vi "Fdx Configure Rx VL Filter.vi"(8 "error in":errorcluster, 9 "VLControl":T1 {"FilterMode" items=["FDX_RX_VL_FLT_DIS", "FDX_RX_VL_FLT_ENA ", "FDX_RX_VL_FLT_ENA_INV"]; "VerificationMode" items=["FDX_RX_VL_CHECK_ENA_DEFAULT"=65535, "FDX_RX_VL_CHECK_REDMAM"=16, "DX_RX_VL_CHECK_TRAFIC"=8, "FDX_RX_VL_CHECK_FRAMESIZE"=4, "FDX_RX_VL_CHECK_SNINTEG"=2, "FDX_RX_VL_CHECK_INVPAC"=1, "FDX_RX_VL_CHECK_DISA"=0]; "PayloadMode" items=["FDX_PAYLOAD_FULL", "FDX_PAYLOAD_IP_EXT", "FDX_PAYLOAD_IP", "FDX_PAYLOAD_MAC"]; "EnableMode" items=["FDX_RX_VL_DIS "=0, "FDX_RX_VL_ENA_STAT"=1, "FDX_RX_VL_ENA_CNT "=2, "FDX_RX_VL_ENA_MON_ALL"=3, "FDX_RX_VL_ENA_MON_GOOD"=7, "FDX_RX_VL_ENA_EXT"=4]}, 11 "InstrumentHandle_port":u32) -> (0 "error out":errorcluster, 3 "InstrumentHandle_port":u32)   [LabVIEW 2020, in "AIM664LV.lvlib"]
doc: "This function is used to control the Virtual link specific setting for a receive port. The settings for a VL can be equivalent to a VL capture filter. That means, only data of a VL which is enabled for capturing, will be stored in the associated buffer."
uses:
  AIM664LV.lvlib
  AFDX_LibraryAdmin/FdxGlobalDllPath.vi
panel:
  # "Inputs"
  # "Outputs"
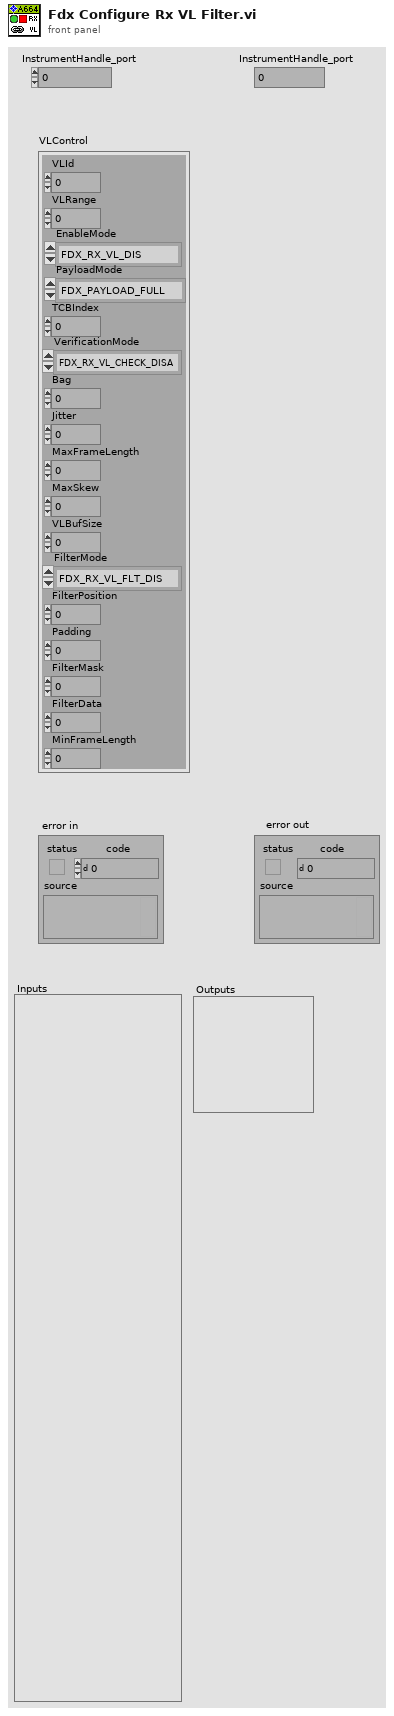
[diagram p1: front panel]
types:
  T1 = cluster{"VLId":u32, "VLRange":u32, "EnableMode":u32, "PayloadMode":u32, "TCBIndex":u32, "VerificationMode":u32, "Bag":u32, "Jitter":u32, "MaxFrameLength":u32, "MaxSkew":u32, "VLBufSize":u32, "FilterMode":u32, "FilterPosition":u32, "Padding":u32, "FilterMask":u32, "FilterData":u32, "MinFrameLength":u32}
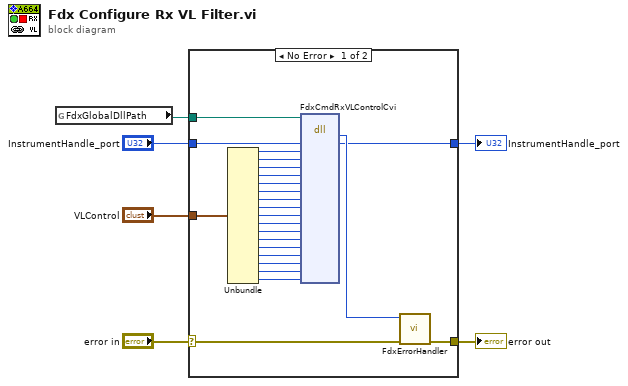
[diagram p0: block diagram]
diagram:
  n1 = global read "FdxGlobalDllPath.vi" "FdxGlobalDllPath"() -> (w4:path)
  n2 = case shown="No Error" "error in" {
    selector: "error in" -> [w29 w32]
    tunnel: [w30 w32] -> w6
    tunnel: w4 -> [w10 _]
    tunnel: "VLControl" -> [w9 _]
    tunnel: "InstrumentHandle_port" -> [w8 w31]
    tunnel: [w7 w31] -> w1
    frame No Error {
      n3 = Unbundle(w9) -> ("VLId"=w27:u32, "VLRange"=w26:u32, "EnableMode"=w25:u32, "PayloadMode"=w24:u32, "TCBIndex"=w23:u32, "VerificationMode"=w22:u32, "Bag"=w21:u32, "Jitter"=w20:u32, "MaxFrameLength"=w19:u32, "MaxSkew"=w18:u32, "VLBufSize"=w17:u32, "FilterMode"=w16:u32, "FilterPosition"=w15:u32, "Padding"=w14:u32, "FilterMask"=w13:u32, "FilterData"=w12:u32, "MinFrameLength"=w11:u32)
      n4 = dll-call lib="aim_fdx.19.dll" fn="FdxCmdRxVLControlCvi"(path in=w10, "InstrumentHandle"=w8, "VLId"=w27, "VLRange"=w26, "EnableMode"=w25, "PayloadMode"=w24, "TCBIndex"=w23, "VerificationMode"=w22, "Bag"=w21, "Jitter"=w20, "MaxFrameLength"=w19, "MaxSkew"=w18, "VLBufSize"=w17, "FilterMode"=w16, "FilterPosition"=w15, "Padding"=w14, "FilterMask"=w13, "FilterData"=w12, "MinFrameLength"=w11) -> ("status"=w28:i32, "InstrumentHandle"=w7:u32)  [unwired: 19 in, 2 out]
      n5 = call "FdxErrorHandler.vi"("error in"=w29, "AIM Error"=w28) -> ("error out"=w30:errorcluster)  [unwired: 9 in]
    }
    frame Error {
    }
  }
  "error out" <- w6
  "InstrumentHandle_port" <- w1
